vi "rs3_RGB_to_Picture6.vi"(0 "RGB array":u8[](array[numeric]), 1 "Color format":enum16{"Monochrome", "RGB internal (RGB)"}(ring), 2 "Transpose":bool, 5 "RGB  X, width":i32, 7 "RGB Y, height":i32, 9 "AWB":bool, 11 "error in (no error)":errorcluster, 12 "White Balance":cluster{"Red":dbl, "Green":dbl, "Blue":dbl}={"Red"=1.0, "Green"=1.0, "Blue"=1.0} {"Blue" format="%_3g"; "Green" format="%_3g"; "Red" format="%_3g"}, 14 "White Balance":bool) -> (6 "new picture":picture, 15 "error out":errorcluster)   [LabVIEW 2017, in "libRealSense3.lvlib"]
doc: "This converts an 1D input array into a 2D picture, and applies some white balance correction if requested."
uses:
  libRealSense3.lvlib
  <vilib>/Analysis/NI_AALBase.lvlib
  <vilib>/Analysis/baseanly.llb/Mean (DBL).vi
panel:
  # "RS3 RGB to Picture"
  # "(C) Intel Corp. 2017,  AGJ"
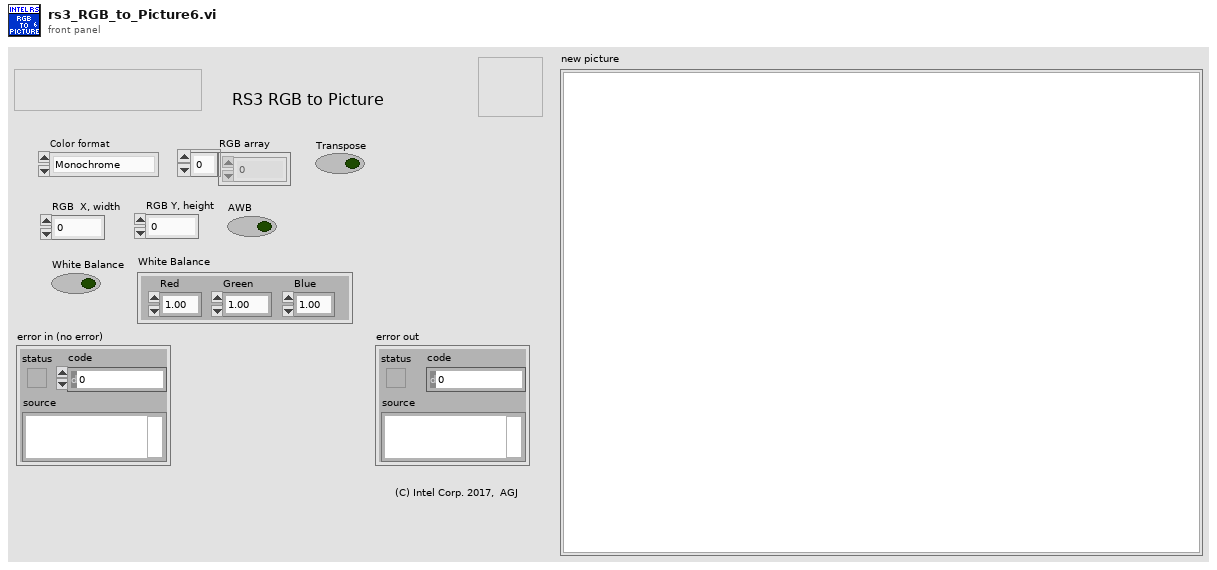
[diagram p1: front panel]
types:
  T1 = typedef "imagedata.ctl" = cluster{"image type":i32, "image depth":i32, "image":u8[], "mask":u8[], "colors":u32[], "Rectangle":cluster{"left":i16, "top":i16, "right":i16, "bottom":i16}}
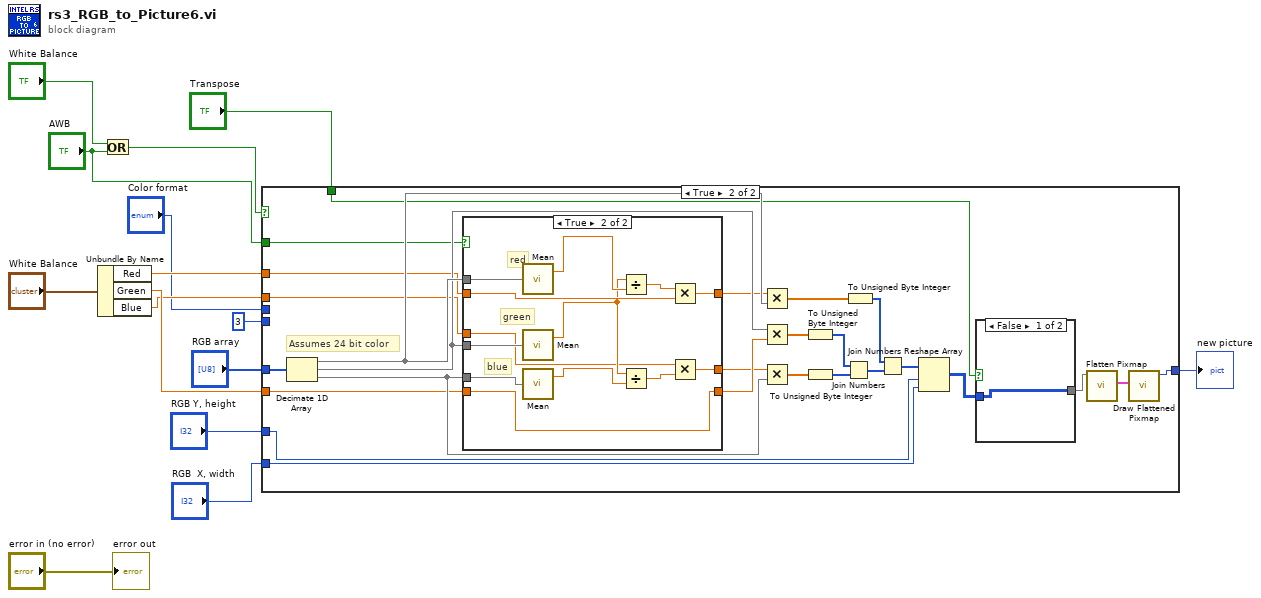
[diagram p0: block diagram]
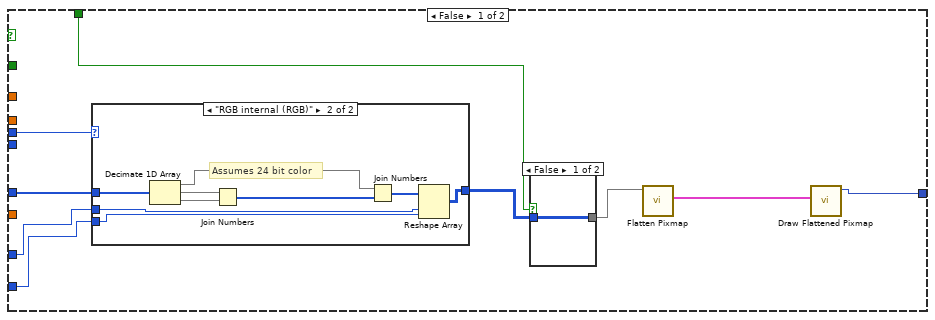
[diagram p2: hidden frame]
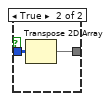
[diagram p3: hidden frame]
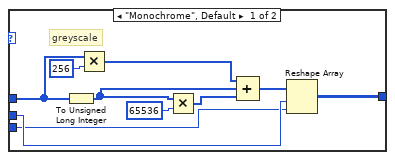
[diagram p4: hidden frame]
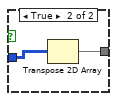
[diagram p5: hidden frame]
diagram:
  n1 = Unbundle By Name("White Balance") -> ("Red"=w10:dbl, "Green"=w9:dbl, "Blue"=w8:dbl)
  n2 = Or(x="White Balance", y="AWB") -> (x .or. y?=w3:bool)
  n3 = case shown="True" w3 {
    tunnel: [w24 w61] -> w15
    tunnel: "RGB array" -> [w23 w69]
    tunnel: "RGB Y, height" -> [w22 w60]
    tunnel: "RGB  X, width" -> [w21 w68]
    tunnel: 3 ("# of bytes/number") -> [_ _]
    tunnel: w10 -> [_ w55]
    tunnel: w9 -> [_ w53]
    tunnel: w8 -> [_ w52]
    tunnel: "AWB" -> [_ w50]
    tunnel: "Color format" -> [w20 _]
    tunnel: "Transpose" -> [w16 w47]
    frame False {
      n4 = case shown="\"RGB internal (RGB)\"" w20 {
        tunnel: [w35 w45] -> w18
        tunnel: w23 -> [w31 w43]
        tunnel: w22 -> [w37 w42]
        tunnel: w21 -> [w36 w41]
        frame "Monochrome", Default {
          # "greyscale"
          n5 = To Unsigned Long Integer(number=w31) -> (unsigned 32bit integer=w28:u32[])
          n6 = Multiply(x=w31, y=u32 256) -> (x*y=w32:u32[])
          n7 = Multiply(x=w28, y=u32 65536) -> (x*y=w30:u32[])
          n8 = Compound Arithmetic op=ADD(w32, w28, w30) -> (w29:u32[])
          n9 = Reshape Array(w29, w37, w36) -> (w35:u32[][])
        }
        frame "RGB internal (RGB)" {
          # "Assumes 24 bit color"
          n10 = Decimate 1D Array(w43) -> (w40:u8[], w39:u8[], w38:u8[])
          n11 = Join Numbers(hi=w39, lo=w38) -> ((hi.lo)=w46:u16[])
          n12 = Join Numbers(hi=w40, lo=w46) -> ((hi.lo)=w44:u32[])
          n13 = Reshape Array(w44, w42, w41) -> (w45:u32[][])
        }
      }
      n14 = case shown="False" w16 {
        tunnel: w18 -> [w25 w27]
        tunnel: [w25 w26] -> w17
        frame False {
        }
        frame True {
          n15 = Transpose 2D Array(2D array=w27) -> (transposed array=w26:u32[][])
        }
      }
      n16 = call <vilib>:"Flatten Pixmap.vi"("24-bit pixmap"=w17) -> ("image data"=w19:T1)  [unwired: 10 in]
      n17 = call <vilib>:"Draw Flattened Pixmap.vi"("image data"=w19) -> ("new picture"=w24:picture)  [unwired: 8 in]
    }
    frame True {
      # "Assumes 24 bit color"
      n18 = Decimate 1D Array(w69) -> (w59:u8[], w58:u8[], w57:u8[])
      n19 = case shown="True" w50 {
        tunnel: w59 -> [_ w91]
        tunnel: w58 -> [_ w90]
        tunnel: w57 -> [_ w89]
        tunnel: [w78 w84] -> w56
        tunnel: w55 -> [w78 w85]
        tunnel: [w77 w79] -> w54
        tunnel: w53 -> [w77 w79]
        tunnel: w52 -> [w76 w81]
        tunnel: [w76 w80] -> w51
        frame False {
        }
        frame True {
          # "blue"
          # "green"
          # "red"
          n20 = call-poly <vilib>:"Mean.vi"("X"=w91) -> ("mean"=w88:dbl)  [unwired: 1 out]
          n21 = call-poly <vilib>:"Mean.vi"("X"=w90) -> ("mean"=w83:dbl)  [unwired: 1 out]
          n22 = call-poly <vilib>:"Mean.vi"("X"=w89) -> ("mean"=w87:dbl)  [unwired: 1 out]
          n23 = Divide(x=w83, y=w88) -> (x/y=w86:dbl)
          n24 = Divide(x=w83, y=w87) -> (x/y=w82:dbl)
          n25 = Multiply(x=w86, y=w85) -> (x*y=w84:dbl)
          n26 = Multiply(x=w81, y=w82) -> (x*y=w80:dbl)
        }
      }
      n27 = Multiply(x=w56, y=w59) -> (x*y=w67:dbl[])
      n28 = Multiply(x=w58, y=w54) -> (x*y=w63:dbl[])
      n29 = Multiply(x=w51, y=w57) -> (x*y=w64:dbl[])
      n30 = To Unsigned Byte Integer(number=w63) -> (unsigned 8bit integer=w65:u8[])
      n31 = To Unsigned Byte Integer(number=w64) -> (unsigned 8bit integer=w62:u8[])
      n32 = Join Numbers(hi=w65, lo=w62) -> ((hi.lo)=w72:u16[])
      n33 = To Unsigned Byte Integer(number=w67) -> (unsigned 8bit integer=w66:u8[])
      n34 = Join Numbers(hi=w66, lo=w72) -> ((hi.lo)=w70:u32[])
      n35 = Reshape Array(w70, w60, w68) -> (w49:u32[][])
      n36 = case shown="False" w47 {
        tunnel: w49 -> [w73 w75]
        tunnel: [w73 w74] -> w48
        frame False {
        }
        frame True {
          n37 = Transpose 2D Array(2D array=w75) -> (transposed array=w74:u32[][])
        }
      }
      n38 = call <vilib>:"Flatten Pixmap.vi"("24-bit pixmap"=w48) -> ("image data"=w71:T1)  [unwired: 10 in]
      n39 = call <vilib>:"Draw Flattened Pixmap.vi"("image data"=w71) -> ("new picture"=w61:picture)  [unwired: 8 in]
    }
  }
  "new picture" <- w15
  "error out" <- "error in (no error)"
